vi "Test Configuration.vi"(8 "error in (no error)":errorcluster) -> (0 "error out":errorcluster)   [LabVIEW 2019]
uses:
  <vilib>/Utility/sysdir.llb/System Directory Type.ctl
  <userlib>/_OpenG.lib/numeric/numeric.llb/Random Number Within Range - I32__ogtk.vi
  <vilib>/addons/_JKI Toolkits/Caraya/classes/Assert/Assert Equal Value_Variant.vi
  <vilib>/addons/_JKI Toolkits/Caraya/classes/Assert/Assert Not Error.vi
  <userlib>/LevyLab/Configuration/Configuration.lvclass
  <vilib>/addons/_JKI Toolkits/Caraya/classes/Assert/Assert.lvclass
  <vilib>/addons/_JKI Toolkits/Caraya/classes/Test/Test.lvclass
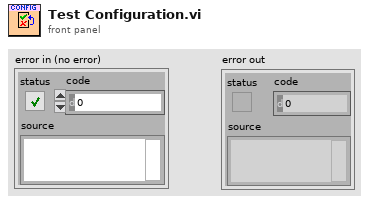
[diagram p1: front panel]
types:
  T1 = typedef "System Directory Type.ctl" = i32
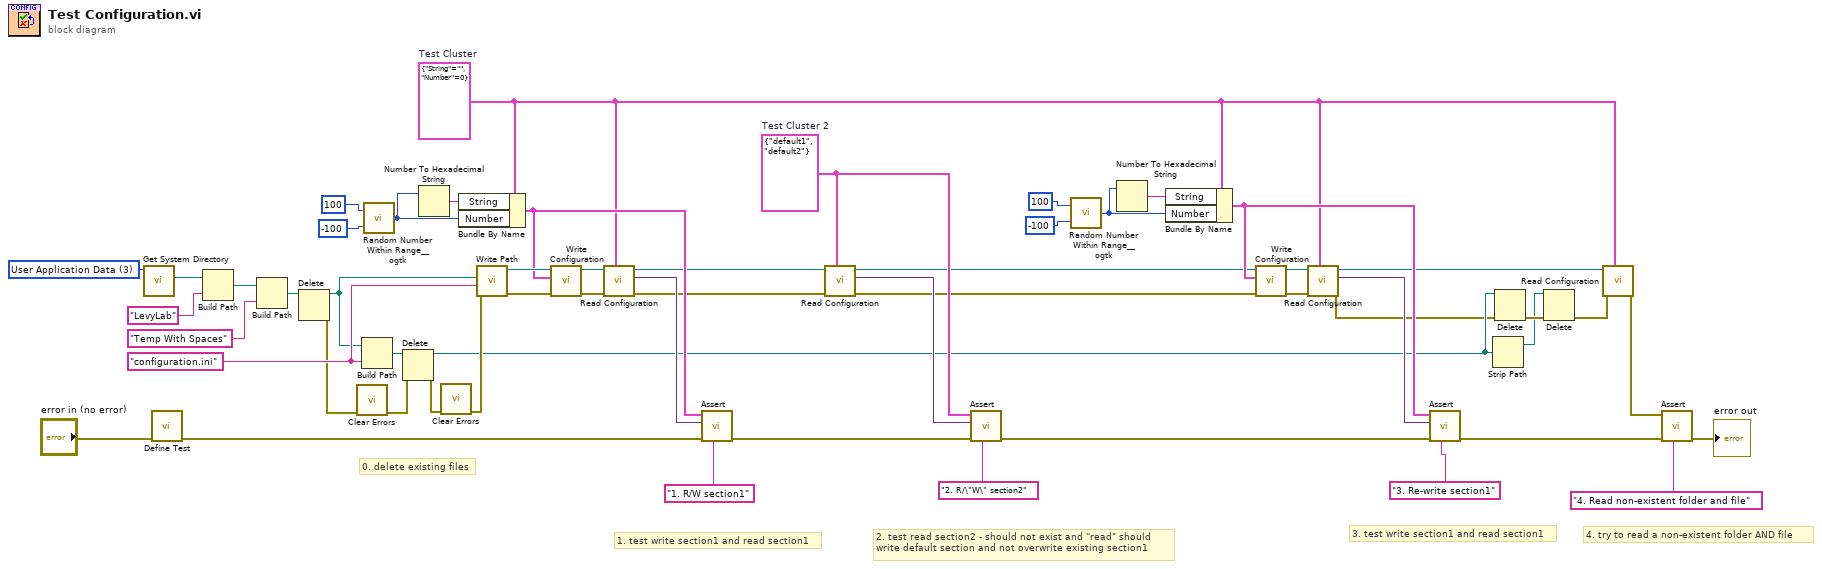
[diagram p0: block diagram]
diagram:
  w9 = "configuration.ini" ("name or relative path")
  w23 = cluster{"String":string, "String 2":string} {"String"="default1", "String 2"="default2"}  # Test Cluster 2
  w49 = T1 3 items=["User Home"=0, "User Desktop"=1, "User Documents"=2, "User Application Data"=3, "User Preferences"=4, "User Temporary"=5, "Public Documents"=6, "Public Application Data"=7, "Public Preferences"=8, "Public Cache"=13, "System Core Libraries"=9, "System Installed Libraries"=10, "Application Files"=11, "Boot Volume Root"=12] ("system directory type")
  w21 = cluster{"String":string, "Number":i32} {"String"="", "Number"=0}  # Test Cluster
  # "4. try to read a non-existent folder AND file"
  # "3. test write section1 and read section1"
  # "0. delete existing files"
  # "2. test read section2 - should not exist and \"read\" should\nwrite default section and not overwrite existing section1"
  # "1. test write section1 and read section1"
  n1 = call <vilib>:"Get System Directory.vi"("system directory type"=w49) -> ("system directory"=w36:path)  [unwired: 10 in]
  n2 = call <vilib>:"Define Test.vi"("error in (no error)"="error in (no error)") -> ("error out"=w19:errorcluster)  [unwired: 9 in, 1 out]
  n3 = Build Path(base path=w36, name or relative path="LevyLab") -> (appended path=w34:path)
  n4 = Build Path(base path=w34, name or relative path="Temp With Spaces") -> (appended path=w8:path)
  n5 = Delete(path (use dialog)=w8) -> (deleted path=w7:path, error out=w6:errorcluster)  [unwired: 4 in, 1 out]
  n6 = call <vilib>:"Clear Errors.vi"("error in (no error)"=w6) -> ("error out"=w5:errorcluster)  [unwired: 5 in, 1 out]
  n7 = Build Path(base path=w7, name or relative path=w9) -> (appended path=w44:path)
  n8 = call-poly <userlib>:"Random Number Within Range__ogtk.vi"("High"=100 ("Number"), "Low"=-100 ("Number")) -> ("Random Number"=w32:i32)  [unwired: 3 in]
  n9 = Delete(path (use dialog)=w44, error in=w5) -> (deleted path=w10:path, error out=w31:errorcluster)  [unwired: 3 in, 1 out]
  n10 = Number To Hexadecimal String(2:w32) -> (0:w50:string)  [unwired: 1 in]
  n11 = call <vilib>:"Clear Errors.vi"("error in (no error)"=w31) -> ("error out"=w20:errorcluster)  [unwired: 5 in, 1 out]
  n12 = Bundle By Name(cluster=w21, "String"=w50, "Number"=w32) -> (w47:cluster{"String":string, "Number":i32})
  n13 = call <userlib>:"Write Path.vi"("error in (no error)"=w20, "Filename [Configuration.ini]"=w9, "Path"=w7) -> ("error out"=w48:errorcluster, "Configuration out"=w55:refnum<class "Configuration.lvclass">)  [unwired: 7 in]
  n14 = call <userlib>:"Write Configuration.vi"("error in (no error)"=w48, "Variant"=w47, "Configuration in"=w55) -> ("error out"=w53:errorcluster, "Configuration out"=w54:refnum<class "Configuration.lvclass">)  [unwired: 7 in]
  n15 = call <userlib>:"Read Configuration.vi"("INI Fomatted Cluster Type"=w21, "error in (no error)"=w53, "Configuration in"=w54) -> ("error out"=w15:errorcluster, "Configuration"=w25:variant, "Configuration out"=w12:refnum<class "Configuration.lvclass">)  [unwired: 6 in]
  n16 = call-poly <vilib>:"Assert.vi"("Label"="1. R/W section1", "error in (no error)"=w19, "Y"=w25, "X"=w47) -> ("error out"=w18:errorcluster)  [unwired: 6 in, 1 out]
  n17 = call <userlib>:"Read Configuration.vi"("INI Fomatted Cluster Type"=w23, "error in (no error)"=w15, "Configuration in"=w12) -> ("error out"=w14:errorcluster, "Configuration"=w24:variant, "Configuration out"=w11:refnum<class "Configuration.lvclass">)  [unwired: 6 in]
  n18 = call-poly <vilib>:"Assert.vi"("Label"="2. R/\"W\" section2", "error in (no error)"=w18, "Y"=w24, "X"=w23) -> ("error out"=w17:errorcluster)  [unwired: 6 in, 1 out]
  n19 = call-poly <userlib>:"Random Number Within Range__ogtk.vi"("High"=100 ("Number"), "Low"=-100 ("Number")) -> ("Random Number"=w43:i32)  [unwired: 3 in]
  n20 = Number To Hexadecimal String(2:w43) -> (0:w42:string)  [unwired: 1 in]
  n21 = Bundle By Name(cluster=w21, "String"=w42, "Number"=w43) -> (w22:cluster{"String":string, "Number":i32})
  n22 = call <userlib>:"Write Configuration.vi"("error in (no error)"=w14, "Variant"=w22, "Configuration in"=w11) -> ("error out"=w13:errorcluster, "Configuration out"=w39:refnum<class "Configuration.lvclass">)  [unwired: 7 in]
  n23 = call <userlib>:"Read Configuration.vi"("INI Fomatted Cluster Type"=w21, "error in (no error)"=w13, "Configuration in"=w39) -> ("error out"=w3:errorcluster, "Configuration"=w38:variant, "Configuration out"=w4:refnum<class "Configuration.lvclass">)  [unwired: 6 in]
  n24 = call-poly <vilib>:"Assert.vi"("Label"="3. Re-write section1", "error in (no error)"=w17, "Y"=w38, "X"=w22) -> ("error out"=w16:errorcluster)  [unwired: 6 in, 1 out]
  n25 = Strip Path(path=w10) -> (stripped path=w28:path)  [unwired: 1 out]
  n26 = Delete(path (use dialog)=w10, error in=w3) -> (error out=w29:errorcluster)  [unwired: 3 in, 2 out]
  n27 = Delete(path (use dialog)=w28, error in=w29) -> (error out=w2:errorcluster)  [unwired: 3 in, 2 out]
  n28 = call <userlib>:"Read Configuration.vi"("INI Fomatted Cluster Type"=w21, "error in (no error)"=w2, "Configuration in"=w4) -> ("error out"=w1:errorcluster)  [unwired: 6 in, 2 out]
  n29 = call-poly <vilib>:"Assert.vi"("Label"="4. Read non-existent folder and file", "error in (no error)"=w16, "Not Error?"=w1) -> ("error out"=→"error out":errorcluster)  [unwired: 7 in, 1 out]
